vi "Autonomous Independent.vi"() -> ()   [LabVIEW 2016]
doc: "This VI is called when autonomous begins, and will automatically be terminated when autonomous ends. You can carry out timed or sensor driven robot movement independently without needing to return to the caller."
uses:
  <vilib>/Rock Robotics/WPI/ThirdParty/CanMotor/TalonSRX/WPI_CANTalonSRX_APIControlMode.ctl
  Auton.ctl
  AutonEncCounts.ctl
  <vilib>/Rock Robotics/WPI/Relay/WPI_RelayValue.ctl
  <vilib>/Rock Robotics/Network Tables/NT Read String.vi
  <vilib>/Rock Robotics/Network Tables/NT Write String.vi
  <vilib>/Rock Robotics/Network Tables/NT Write Number.vi
panel:
  out "ElapsedTime":u32
  # "Be sure to right-click and choose Data Operations>>Make Current Value default if you want to save the array values with the VI"
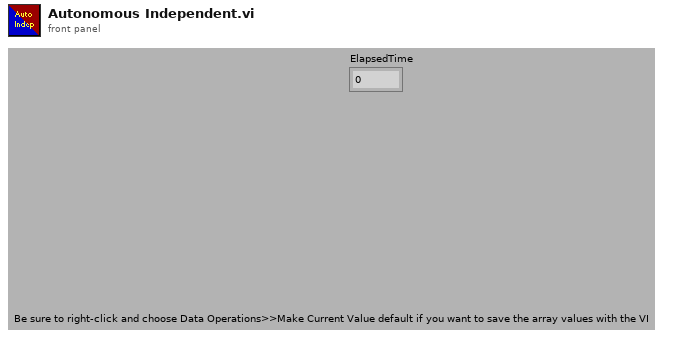
[diagram p1: front panel]
types:
  T1 = enum16{"Integer", "Float", "Boolean", "Enum", "String", "Close"}
  T2 = typedef "Auton.ctl" = enum16{"VisionTarget", "Wait", "Initialize", "Stop", "Reset", "StraightForward", "StraightBack", "SolenoidControl", "SharpLeftCurve", "SharpRightCurve", "GradLeftCurve", "GradRightCurve", "TurnLeft90", "TurnRight90", "TurnLeft60", "TurnRight60", "TurnLeft45", "TurnRight45", "Shoot", "SpinUp", "GearApproach", "ShortShoot", "SlowForward", "TimeForward", "Pause", "HopperDrive"}
  T3 = typedef "AutonEncCounts.ctl" = i32
  T4 = cluster{"Action":T2[], "EncoderCounts":T3[], "GearLift":bool[], "FuelFlap":bool[]}
  T5 = cluster{"Action":T2[], T3[], "GearLift":bool[], "FuelFlap":bool[]}
  T6 = typedef "WPI_MotorControlDeviceRef.ctl" = cluster{"DeviceStatus":errorcluster, "Type":T7, "PWM":cluster{"PWM Channel":T8, "DeadBand":T9}, "CAN":cluster{"Device Number":u8, "SetOutput VI Ref":variant, "GetOutput VI Ref":variant, "Enable VI Ref":variant, "Disable VI Ref":variant, "Data":variant}, "Invert":bool}
  T7 = typedef "WPI_MotorControlType.ctl" = enum16{"PWM", "CAN"}
  T8 = typedef "FPGA_DIOPWMChannel.ctl" = enum8{"PWM 0", "PWM 1", "PWM 2", "PWM 3", "PWM 4", "PWM 5", "PWM 6", "PWM 7", "PWM 8", "PWM 9", "PWM MXP 0", "PWM MXP 1", "PWM MXP 2", "PWM MXP 3", "PWM MXP 4", "PWM MXP 5", "PWM MXP 6", "PWM MXP 7", "PWM MXP 8", "PWM MXP 9", "Invalid"}
  T9 = typedef "WPI_PWMDeadband.ctl" = cluster{"Name":string, "maxPositivePwm":i32, "minPositivePwm":i32, "centerPwm":i32, "maxNegativePwm":i32, "minNegativePwm":i32, "angularRange":u16}
  T10 = enum16{"Integer", "Float", "Boolean", "Enum", "String"}
  T11 = typedef "WPI_CANTalonSRX_APIControlMode.ctl" = enum8{"Percent VBus", "Speed", "Position", "Slave", "Unchanged / Invalid", "Voltage Compensation", "Current", "Motion Profile", "Motion Magic"}
  T12 = typedef "WPI_RelayValue.ctl" = enum16{"Off", "On", "Forward", "Reverse"}
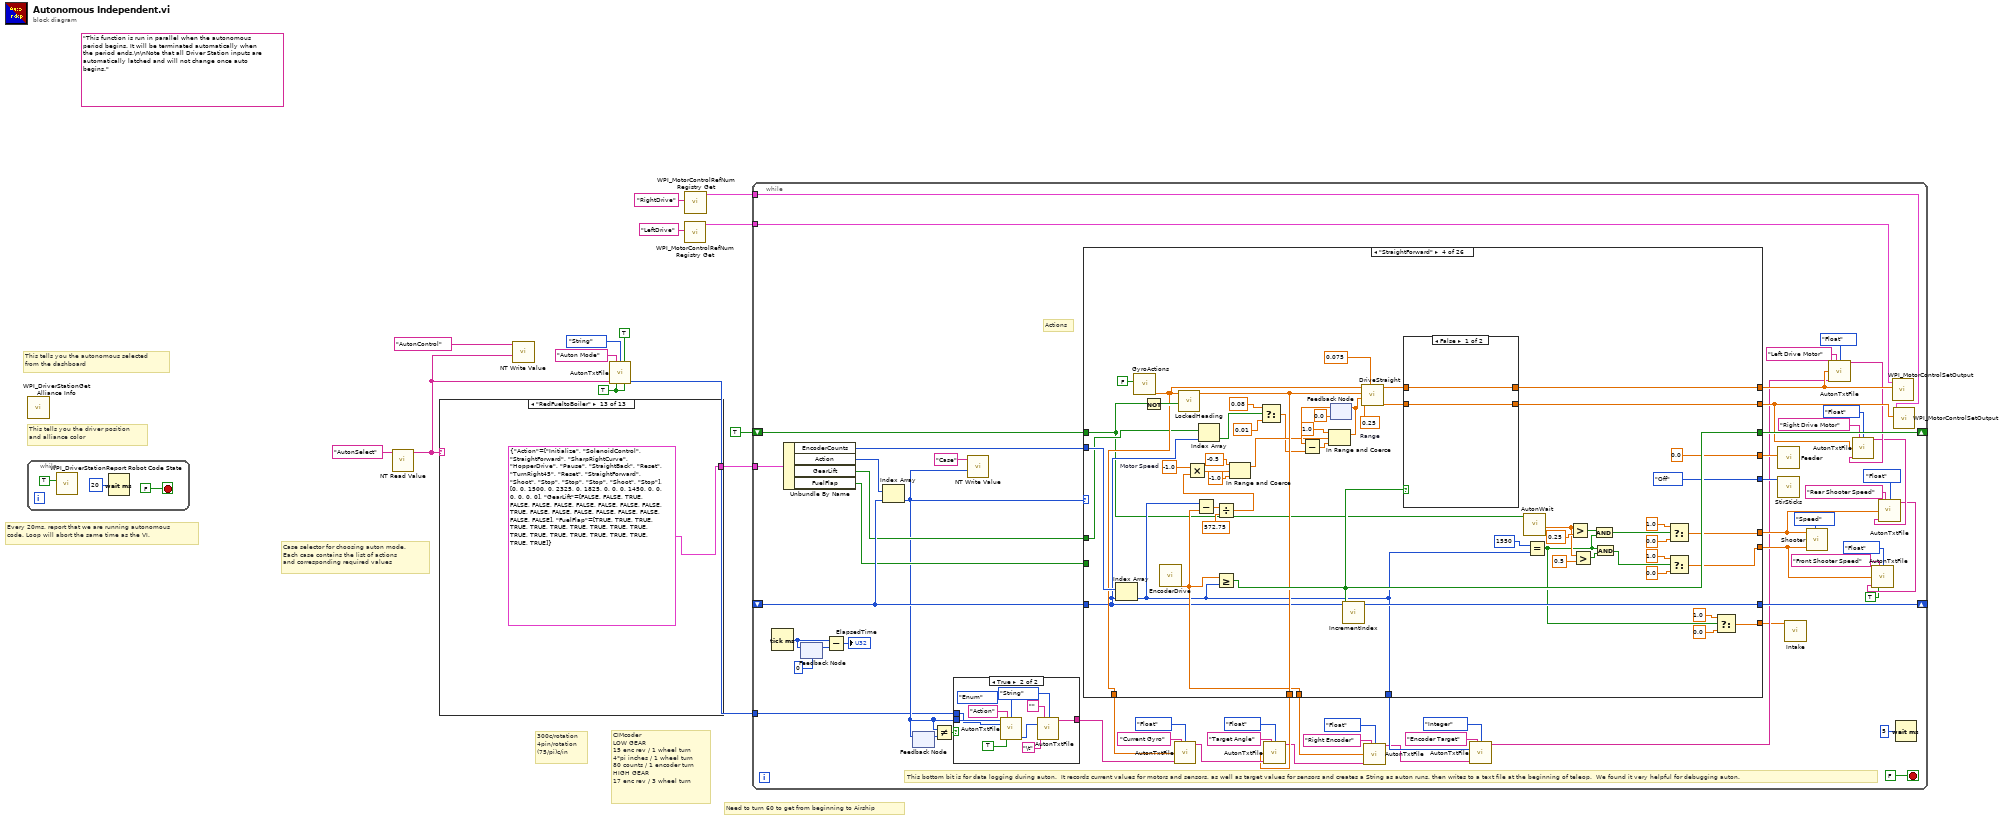
[diagram p0: block diagram]
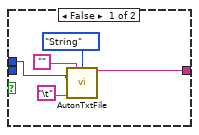
[diagram p2: hidden frame]
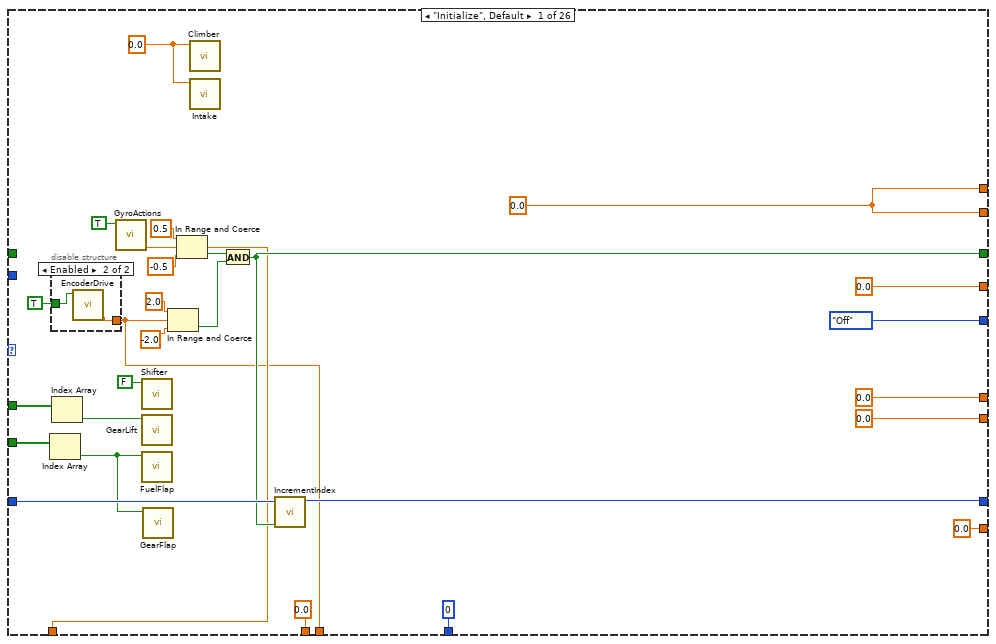
[diagram p3: hidden frame]
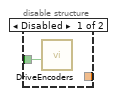
[diagram p4: hidden frame]
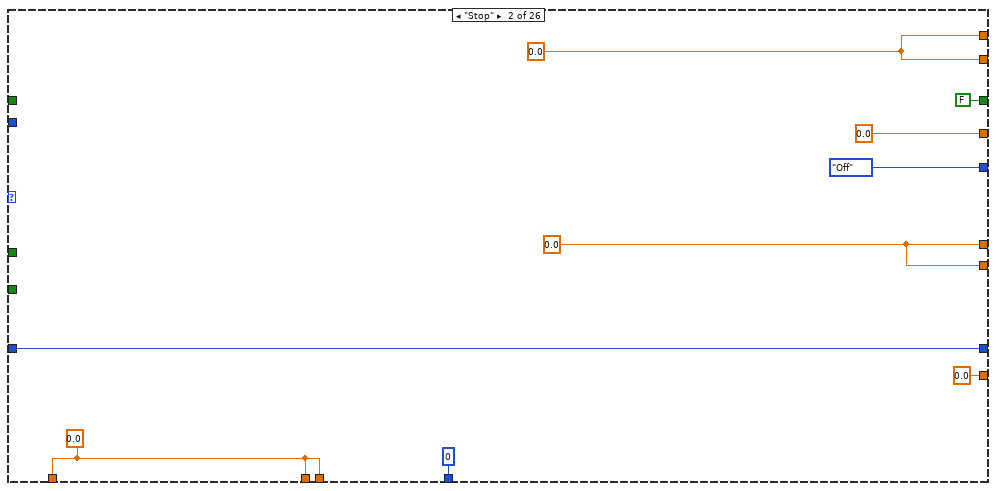
[diagram p5: hidden frame]
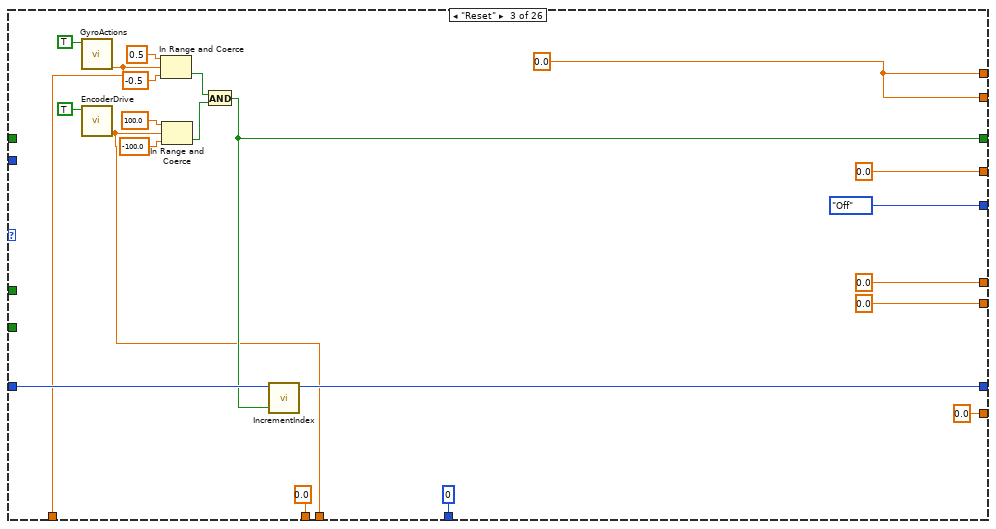
[diagram p6: hidden frame]
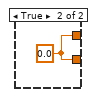
[diagram p7: hidden frame]
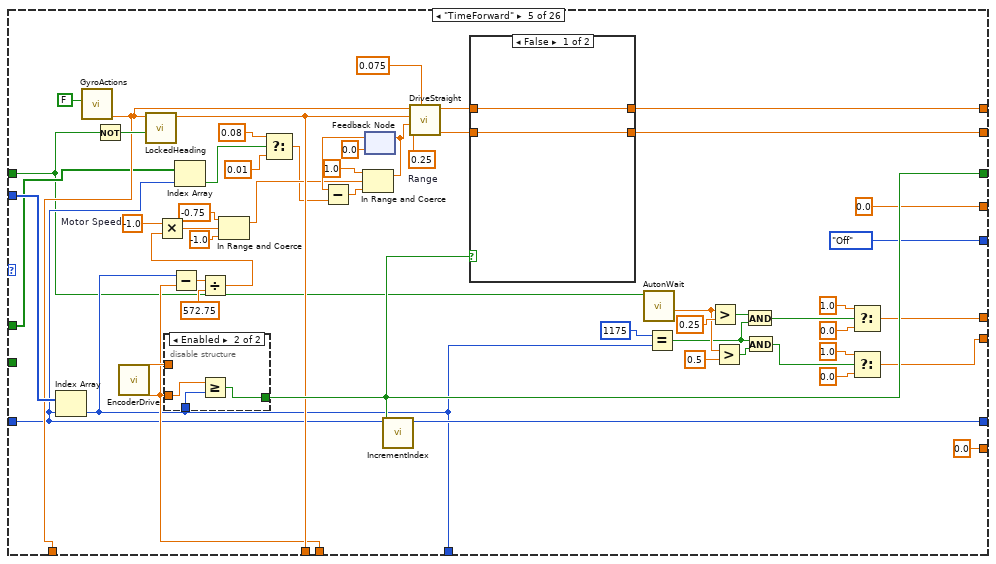
[diagram p8: hidden frame]
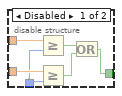
[diagram p9: hidden frame]
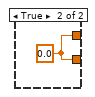
[diagram p10: hidden frame]
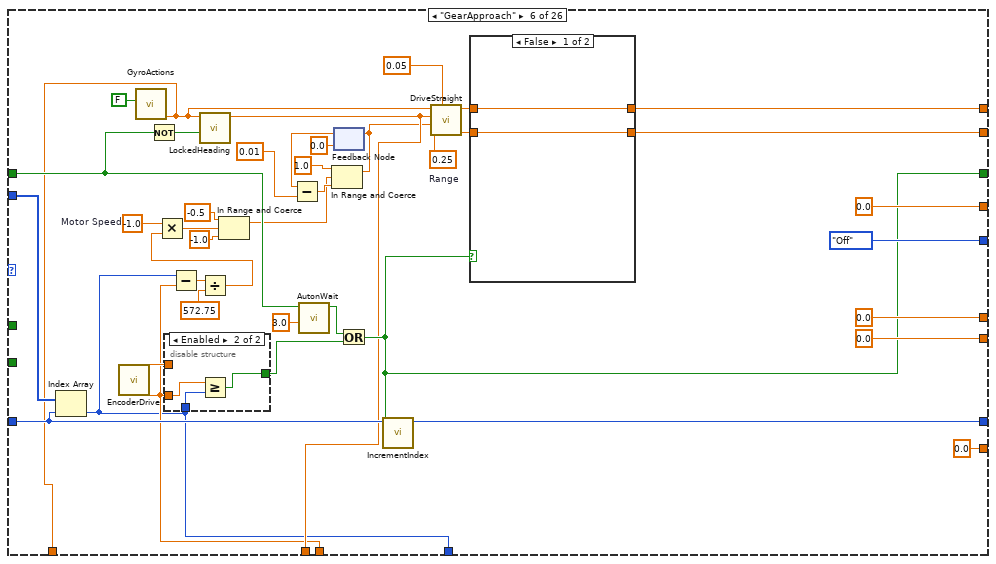
[diagram p11: hidden frame]
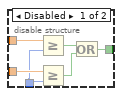
[diagram p12: hidden frame]
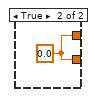
[diagram p13: hidden frame]
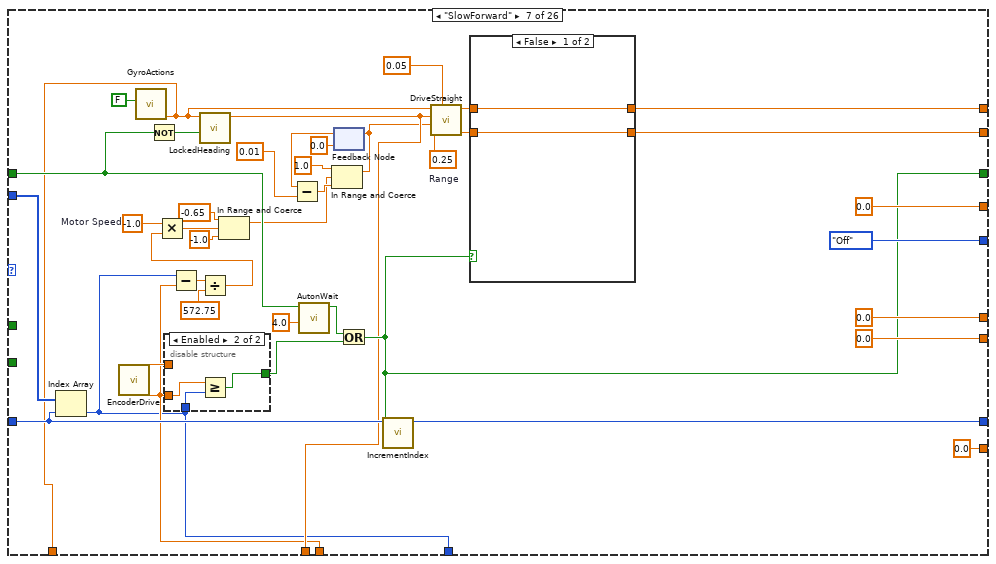
[diagram p14: hidden frame]
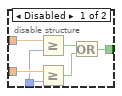
[diagram p15: hidden frame]
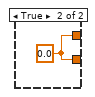
[diagram p16: hidden frame]
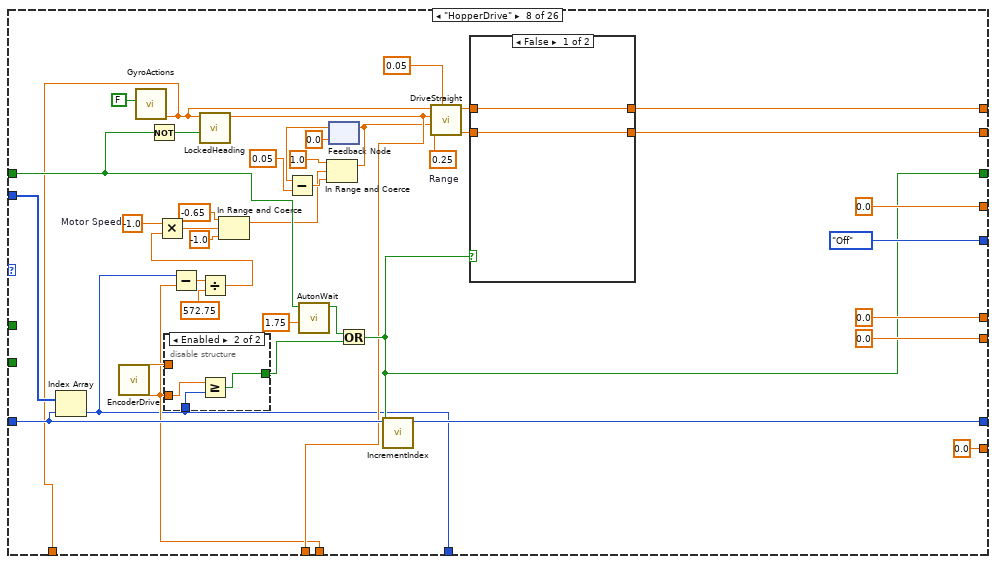
[diagram p17: hidden frame]
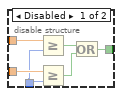
[diagram p18: hidden frame]
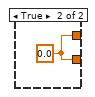
[diagram p19: hidden frame]
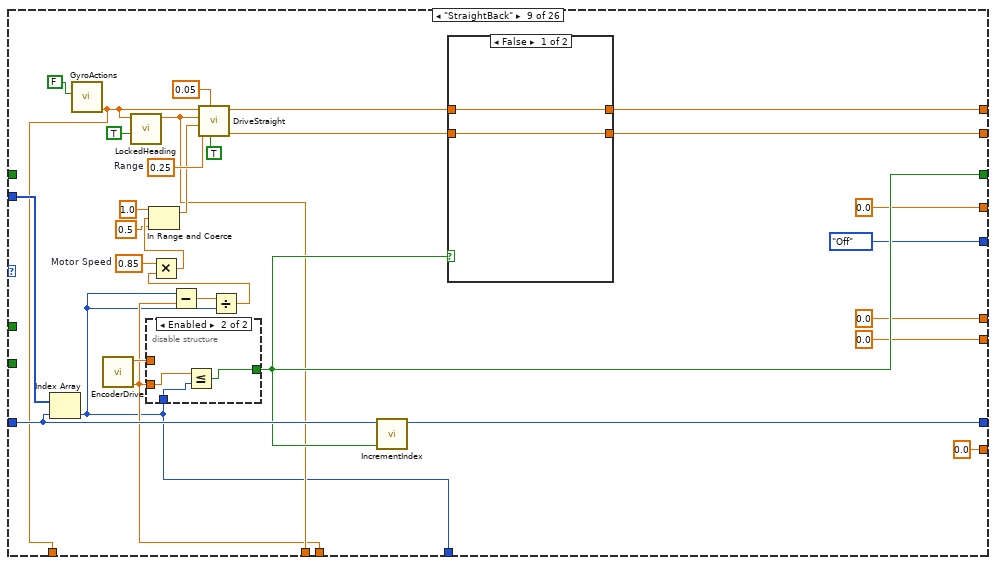
[diagram p20: hidden frame]
diagram:
  w4 = TRUE ("writeToFile?")
  (unwired) "This function is run in parallel when the autonomous period begins. It will be terminated automatically when the period ends.\n\nNote that all Driver Station inputs are automatically latched and will not change once auto begins."
  # "Case selector for choosing auton mode.\nEach case contains the list of actions\nand corresponding required values"
  # "300c/rotation\n4pin/rotation\n(75/pi)c/in"
  # "CIMcoder\nLOW GEAR\n15 enc rev / 1 wheel turn\n4*pi inches / 1 wheel turn\n80 counts / 1 encoder turn\nHIGH GEAR\n17 enc rev / 3 wheel turn"
  # "Need to turn 60 to get from beginning to Airship"
  # "This tells you the autonomous selected\nfrom the dashboard"
  # "Every 20ms, report that we are running autonomous\ncode. Loop will abort the same time as the VI."
  # "This tells you the driver position\nand alliance color"
  n1 = while {
    stop <- FALSE stop-if-true
    n2 = call <vilib>:"WPI_DriverStationReport Robot Code State.vi"("Autonomous"=TRUE) -> ()  [unwired: 10 in, 1 out]
    n3 = Wait (ms)(milliseconds to wait=u32 20) -> ()  [unwired: 1 out]
  }
  n4 = call <vilib>:"WPI_DriverStationGet Alliance Info.vi"() -> ()  [unwired: 12 out]
  n5 = call-poly <vilib>:"NT Read Value.vi"("Name"="AutonSelect") -> ("String"=w2:string)  [unwired: 9 in, 1 out]
  n6 = case shown="\"RedFueltoBoiler\"" w2 {
    tunnel: [T4 {"Action"=[enum."Stop", enum."StraightForward", enum."StraightBack", enum."TurnLeft90", enum."Reset", enum."TurnRight60", enum."TurnRight60", enum."TurnLeft90"], "EncoderCounts"=[0, 0, 0, 0, 0, 0, 0, 0], "GearLift"=[FALSE, TRUE, TRUE, TRUE, TRUE, TRUE, TRUE, TRUE, TRUE, TRUE, TRUE], "FuelFlap"=[FALSE, TRUE, TRUE, TRUE, TRUE, TRUE, TRUE, TRUE, TRUE, TRUE, TRUE]} T4 {"Action"=[enum."Initialize", enum."StraightForward", enum."Stop", enum."TurnLeft90", enum."Reset", enum."TurnRight60", enum."TurnRight60", enum."TurnLeft90"], "EncoderCounts"=[0, 2291, 0, 0, 0, 0, 0, 0], "GearLift"=[FALSE, FALSE, FALSE, TRUE, TRUE, TRUE, TRUE, TRUE, TRUE, TRUE, TRUE], "FuelFlap"=[FALSE, FALSE, FALSE, TRUE, TRUE, TRUE, TRUE, TRUE, TRUE, TRUE, TRUE]} T4 {"Action"=[enum."Initialize", enum."ShortShoot", enum."Reset", enum."TurnRight90", enum."StraightForward", enum."Stop", enum."TurnRight60", enum."TurnLeft90"], "EncoderCounts"=[0, 0, 0, 0, 2500, 0, 0, 0], "GearLift"=[FALSE, FALSE, FALSE, FALSE, FALSE, FALSE, TRUE, TRUE, TRUE, TRUE, TRUE], "FuelFlap"=[FALSE, FALSE, FALSE, FALSE, FALSE, FALSE, FALSE, FALSE, TRUE, TRUE, TRUE]} T4 {"Action"=[enum."Initialize", enum."ShortShoot", enum."Reset", enum."TurnLeft90", enum."StraightForward", enum."Stop", enum."TurnRight60", enum."TurnLeft90"], "EncoderCounts"=[0, 0, 0, 0, 2500, 0, 0, 0], "GearLift"=[FALSE, FALSE, FALSE, FALSE, FALSE, FALSE, TRUE, TRUE, TRUE, TRUE, TRUE], "FuelFlap"=[FALSE, FALSE, FALSE, FALSE, FALSE, FALSE, FALSE, FALSE, TRUE, TRUE, TRUE]} T4 {"Action"=[enum."Initialize", enum."SpinUp", enum."Shoot", enum."Stop", enum."StraightForward", enum."Stop", enum."TurnRight60", enum."TurnLeft90"], "EncoderCounts"=[0, 0, 0, 0, 0, 0, 0, 0], "GearLift"=[FALSE, FALSE, FALSE, FALSE, TRUE, TRUE, TRUE, TRUE, TRUE, TRUE, TRUE], "FuelFlap"=[FALSE, FALSE, FALSE, FALSE, FALSE, FALSE, FALSE, FALSE, TRUE, TRUE, TRUE]} T4 {"Action"=[enum."Initialize", enum."StraightForward", enum."Reset", enum."TurnLeft60", enum."Reset", enum."GearApproach", enum."SolenoidControl", enum."Pause", enum."StraightBack", enum."Reset", enum."TurnRight60", enum."Reset", enum."StraightForward", enum."Stop"], "EncoderCounts"=[0, 1550, 0, 0, 0, 1650, 0, 0, 500, 0, 0, 0, 7000, 0], "GearLift"=[FALSE, FALSE, FALSE, FALSE, FALSE, FALSE, TRUE, FALSE, FALSE, FALSE, FALSE, FALSE, FALSE, FALSE], "FuelFlap"=[FALSE, FALSE, FALSE, FALSE, FALSE, FALSE, FALSE, FALSE, FALSE, FALSE, FALSE, FALSE, FALSE, FALSE]} T4 {"Action"=[enum."Initialize", enum."StraightForward", enum."Reset", enum."TurnRight60", enum."Reset", enum."StraightForward", enum."SolenoidControl", enum."Pause", enum."StraightBack", enum."Reset", enum."TurnLeft60", enum."Reset", enum."StraightForward", enum."Stop"], "EncoderCounts"=[0, 1550, 0, 0, 0, 1650, 0, 0, 500, 0, 0, 0, 7000, 0], "GearLift"=[FALSE, FALSE, FALSE, FALSE, FALSE, FALSE, TRUE, FALSE, FALSE, FALSE, FALSE, FALSE, FALSE, FALSE], "FuelFlap"=[FALSE, FALSE, FALSE, FALSE, FALSE, FALSE, FALSE, FALSE, FALSE, FALSE, FALSE, FALSE, FALSE, FALSE]} T4 {"Action"=[enum."Initialize", enum."SlowForward", enum."SolenoidControl", enum."Pause", enum."StraightBack", enum."Stop", enum."TurnRight60", enum."TurnLeft90"], "EncoderCounts"=[0, 1650, 0, 0, 1000, 0, 0, 0], "GearLift"=[FALSE, FALSE, TRUE, FALSE, FALSE, FALSE, TRUE, TRUE, TRUE, TRUE, TRUE], "FuelFlap"=[FALSE, FALSE, FALSE, FALSE, FALSE, FALSE, TRUE, TRUE, TRUE, TRUE, TRUE]} T4 {"Action"=[enum."Initialize", enum."StraightForward", enum."Reset", enum."TurnRight60", enum."Reset", enum."GearApproach", enum."SolenoidControl", enum."Pause", enum."StraightBack", enum."Reset", enum."TurnLeft60", enum."Reset", enum."StraightForward", enum."Stop"], "EncoderCounts"=[0, 1550, 0, 0, 0, 1845, 0, 0, 929, 0, 0, 0, 7000, 0], "GearLift"=[FALSE, FALSE, FALSE, FALSE, FALSE, FALSE, TRUE, FALSE, FALSE, FALSE, FALSE, FALSE, FALSE], "FuelFlap"=[FALSE, FALSE, FALSE, FALSE, FALSE, FALSE, FALSE, FALSE, FALSE, FALSE, FALSE, FALSE, FALSE]} T4 {"Action"=[enum."Initialize", enum."StraightForward", enum."Reset", enum."TurnLeft60", enum."Reset", enum."StraightForward", enum."SolenoidControl", enum."StraightBack", enum."Reset", enum."TurnRight60", enum."Reset", enum."StraightForward", enum."Stop"], "EncoderCounts"=[0, 1471, 0, 0, 0, 1645, 0, 929, 0, 0, 0, 7000, 0], "GearLift"=[FALSE, FALSE, FALSE, FALSE, FALSE, FALSE, TRUE, FALSE, FALSE, FALSE, FALSE, FALSE, FALSE, FALSE], "FuelFlap"=[FALSE, FALSE, FALSE, FALSE, FALSE, FALSE, FALSE, FALSE, FALSE, FALSE, FALSE, FALSE, FALSE]} T5 {"Action"=[enum."Initialize", enum."SolenoidControl", enum."StraightForward", enum."SharpLeftCurve", enum."HopperDrive", enum."Pause", enum."StraightBack", enum."Reset", enum."TurnLeft45", enum."Reset", enum."StraightForward", enum."Shoot", enum."Stop", enum."Stop", enum."Stop", enum."Shoot", enum."Stop"], [0, 0, 1500, 0, 3475, 0, 2935, 0, 0, 0, 1450, 0, 0, 0, 0, 0, 0], "GearLift"=[FALSE, FALSE, TRUE, FALSE, FALSE, FALSE, FALSE, FALSE, FALSE, FALSE, TRUE, FALSE, FALSE, FALSE, FALSE, FALSE, FALSE, FALSE, FALSE], "FuelFlap"=[TRUE, TRUE, TRUE, TRUE, TRUE, TRUE, TRUE, TRUE, TRUE, TRUE, TRUE, TRUE, TRUE, TRUE, TRUE, TRUE, TRUE, TRUE, TRUE]} T4 {"Action"=[enum."Initialize", enum."TimeForward", enum."Stop", enum."TurnLeft90", enum."Reset", enum."TurnRight60", enum."TurnRight60", enum."TurnLeft90"], "EncoderCounts"=[0, 0, 0, 0, 0, 0, 0, 0], "GearLift"=[FALSE, FALSE, FALSE, TRUE, TRUE, TRUE, TRUE, TRUE, TRUE, TRUE, TRUE], "FuelFlap"=[FALSE, FALSE, FALSE, TRUE, TRUE, TRUE, TRUE, TRUE, TRUE, TRUE, TRUE]} T5 {"Action"=[enum."Initialize", enum."SolenoidControl", enum."StraightForward", enum."SharpRightCurve", enum."HopperDrive", enum."Pause", enum."StraightBack", enum."Reset", enum."TurnRight45", enum."Reset", enum."StraightForward", enum."Shoot", enum."Stop", enum."Stop", enum."Stop", enum."Shoot", enum."Stop"], [0, 0, 1500, 0, 2325, 0, 1825, 0, 0, 0, 1450, 0, 0, 0, 0, 0, 0], "GearLift"=[FALSE, FALSE, TRUE, FALSE, FALSE, FALSE, FALSE, FALSE, FALSE, FALSE, TRUE, FALSE, FALSE, FALSE, FALSE, FALSE, FALSE, FALSE, FALSE], "FuelFlap"=[TRUE, TRUE, TRUE, TRUE, TRUE, TRUE, TRUE, TRUE, TRUE, TRUE, TRUE, TRUE, TRUE, TRUE, TRUE, TRUE, TRUE, TRUE, TRUE]}] -> w11
    frame "DoNothing", Default {
    }
    frame "CrossLine" {
    }
    frame "BlueShootAndCross" {
    }
    frame "RedShootAndCross" {
    }
    frame "JustShoot" {
    }
    frame "BlueGearRight" {
      # "603"
    }
    frame "RedGearLeft" {
    }
    frame "GearStraight" {
    }
    frame "BlueGearLeft" {
    }
    frame "RedGearRight" {
    }
    frame "BlueFueltoBoiler" {
    }
    frame "TimedForward" {
    }
    frame "RedFueltoBoiler" {
    }
  }
  n7 = call-poly <vilib>:"NT Write Value.vi"("String"=w2, "Name"="AutonControl") -> ()  [unwired: 9 in, 1 out]
  n8 = call "AutonTxtFile.vi"("dataName"="Auton Mode", "mode"=T1."String", "reset?"=TRUE, "string"=w2, "newLine?"=w4, "doubleSpace?"=w4) -> ("flowControl2"=w1:i32)  [unwired: 8 in, 1 out]
  n9 = call <vilib>:"WPI_MotorControlRefNum Registry Get.vi"("refnum name"="LeftDrive") -> ("MotorControlDevRef"=w10:T6)  [unwired: 9 in, 1 out]
  n10 = call <vilib>:"WPI_MotorControlRefNum Registry Get.vi"("refnum name"="RightDrive") -> ("MotorControlDevRef"=w9:T6)  [unwired: 9 in, 1 out]
  n11 = while {
    shift-right: [w87] -> _
    shift-left: _ -> [w86]
    shift-right: [w84] -> _
    shift-left: TRUE -> [w85]
    tunnel: w11 -> [w76]
    tunnel: w10 -> [w75]
    tunnel: w9 -> [w74]
    tunnel: w1 -> [w33]
    stop <- FALSE stop-if-true
    # "This bottom bit is for data logging during auton.  It records current values for motors and sensors, as well as target values for sensors and creates a String as auton runs, then writes to a text file at the beginning of teleop.  We found it very helpful for debugging auton."
    # "Actions"
    n12 = Tick Count (ms)() -> (millisecond timer value=w72:u32)
    n13 = Unbundle By Name(w76) -> ("EncoderCounts"=w81:T3[], "Action"=w80:T2[], "GearLift"=w83:bool[], "FuelFlap"=w82:bool[])
    n14 = feedback-in #1(w72) -> ()
    n15 = feedback #1(u32 0 ("millisecond timer value")) -> (w73:u32)
    n16 = Subtract(x=w72, y=w73) -> (x-y=→"ElapsedTime":u32)
    n17 = Index Array(array=w80, index=w86) -> (element=w67:T2)
    n18 = feedback-in #2(w67) -> ()
    n19 = feedback #2() -> (w68:T2)  [unwired: 1 in]
    n20 = Not Equal?(x=w67, y=w68) -> (x != y?=w66:bool)
    n21 = case shown="True" w66 {
      tunnel: w67 -> [_ w102]
      tunnel: [w91 w99] -> w32
      tunnel: w33 -> [w90 w100]
      frame False {
        n22 = call "AutonTxtFile.vi"("dataName"="", "mode"=T10."String", "integer"=w90, "string"="\t") -> ("flowControl"=w91:string)  [unwired: 10 in, 1 out]
      }
      frame True {
        n23 = call "AutonTxtFile.vi"("enum"=w102, "dataName"="Action", "mode"=T10."Enum", "integer"=w100, "newLine?"=TRUE) -> ("flowControl2"=w98:i32)  [unwired: 9 in, 1 out]
        n24 = call "AutonTxtFile.vi"("dataName"="", "mode"=T10."String", "integer"=w98, "string"="\t") -> ("flowControl"=w99:string)  [unwired: 10 in, 1 out]
      }
    }
    n25 = call-poly <vilib>:"NT Write Value.vi"("Numeric"=w67, "Name"="Case") -> ()  [unwired: 9 in, 1 out]
    n26 = case shown="\"StraightForward\"" w67 {
      tunnel: [w130 w142 w162 w219 w276 w328 w380 w432 w472 w501 w513 w526 w538 w556 w580 w598 w612 w628 w646 w664 w682 w698 w714 w725 w740 w838] -> w87
      tunnel: [w110 w143 w164 w194 w250 w292 w344 w395 w465 w497 w509 w522 w536 0.0 ("Power") w572 w590 w608 w626 w644 w662 w684 w700 w716 w723 w746 w836] -> w63
      tunnel: [w110 w143 w164 w191 w247 w291 w343 w394 w464 w497 w509 w522 w535 w554 w571 0.0 ("Power") w607 w625 w643 w661 w684 w700 w716 w723 w745 w836] -> w60
      tunnel: w81 -> [_ _ _ w216 w273 w325 w377 w429 w471 _ _ _ _ _ _ _ _ _ _ _ _ _ _ _ _ w831]
      tunnel: w86 -> [w131 w142 w163 w184 w240 w324 w376 w428 w470 w496 w514 w527 w539 w557 w579 w597 w613 w629 w647 w665 w683 w699 w715 w726 w741 w830]
      tunnel: w85 -> [_ _ _ w179 w235 w299 w351 w403 _ w495 w512 w525 w540 w558 w581 w599 w611 w630 w648 w666 w680 w696 w712 w728 w739 w839]
      tunnel: [w111 FALSE ("Completed") w153 w213 w269 w300 w352 w404 w463 w495 w512 w525 w541 w559 w578 w596 w610 w631 w649 w667 w679 w691 w711 w724 w742 w837] -> w84
      tunnel: w83 -> [w129 _ _ w185 w241 _ _ _ _ w500 _ _ _ _ _ _ _ _ _ _ _ _ _ _ _ _]
      tunnel: w82 -> [w128 _ _ _ _ _ _ _ _ w499 _ _ _ _ _ _ _ _ _ _ _ _ _ _ _ _]
      tunnel: [0.0 ("RearMotorIn") w141 0.0 ("RearMotorIn") w186 w242 0.0 ("RearMotorIn") 0.0 ("RearMotorIn") 0.0 ("RearMotorIn") 0.0 ("RearMotorIn") 0.0 ("RearMotorIn") w507 w520 w534 w553 w570 w589 w606 w624 w642 w660 1.0 ("f") 0.8 ("RearMotorIn") w710 w722 0.8 ("RearMotorIn") w824] -> w53
      tunnel: [0.0 ("RearMotorIn") w141 0.0 ("RearMotorIn") w169 w224 0.0 ("RearMotorIn") 0.0 ("RearMotorIn") 0.0 ("RearMotorIn") 0.0 ("RearMotorIn") 0.0 ("RearMotorIn") w507 w520 w534 w553 w570 w589 w606 w624 w642 w660 0.95 ("RearMotorIn") 0.95 ("RearMotorIn") w710 w722 0.95 ("RearMotorIn") w824] -> w51
      tunnel: [0.0 ("Power") 0.0 ("Power") 0.0 ("Power") 0.0 ("Power") 0.0 ("Power") 0.0 ("Power") 0.0 ("Power") 0.0 ("Power") 0.0 ("Power") 0.0 ("Power") w507 w520 w534 w553 w570 w589 w606 w624 w642 w660 1.0 ("RearMotorIn") w695 0.0 ("Power") 0.0 ("RearMotorIn") w744 0.0 ("Power")] -> w78
      tunnel: [WPI_RelayValue."Off" ("RelayValue") WPI_RelayValue."Off" ("RelayValue") WPI_RelayValue."Off" ("RelayValue") WPI_RelayValue."Off" ("RelayValue") WPI_RelayValue."Off" ("RelayValue") WPI_RelayValue."Off" ("RelayValue") WPI_RelayValue."Off" ("RelayValue") WPI_RelayValue."Off" ("RelayValue") WPI_RelayValue."Off" ("RelayValue") WPI_RelayValue."Off" ("RelayValue") WPI_RelayValue."Off" ("RelayValue") WPI_RelayValue."Off" ("RelayValue") WPI_RelayValue."Off" ("RelayValue") WPI_RelayValue."Off" ("RelayValue") WPI_RelayValue."Off" ("RelayValue") WPI_RelayValue."Off" ("RelayValue") WPI_RelayValue."Off" ("RelayValue") WPI_RelayValue."Off" ("RelayValue") WPI_RelayValue."Off" ("RelayValue") WPI_RelayValue."Off" ("RelayValue") WPI_RelayValue."Forward" ("RelayValue") w694 WPI_RelayValue."Off" ("RelayValue") WPI_RelayValue."Off" ("RelayValue") w743 WPI_RelayValue."Off" ("RelayValue")] -> w77
      tunnel: [w109 w137 w148 w196 w252 w297 w349 w401 w450 w489 w505 w518 w532 w551 w568 w587 w604 w622 w640 w658 w674 w687 w707 w719 w733 w833] -> w48
      tunnel: [w108 w137 w147 w195 w251 w295 w347 w399 w448 w489 w504 w517 0.0 ("Yaw") 0.0 ("Yaw") 0.0 ("Yaw") 0.0 ("Yaw") 0.0 ("Yaw") 0.0 ("Yaw") 0.0 ("Yaw") 0.0 ("Yaw") w674 w687 w707 w719 0.0 ("Yaw") w833] -> w45
      tunnel: [0.0 ("LockedHeading") w137 0.0 ("LockedHeading") w197 w253 w296 w348 w400 w449 w489 w504 w517 w531 w550 w567 w586 w603 w621 w639 w657 w674 w687 w707 w719 w732 w833] -> w39
      tunnel: [T3 0 ("EncCounts") T3 0 ("EncCounts") T3 0 ("EncCounts") w190 w246 w294 w346 w398 w447 T3 0 ("EncCounts") T3 0 ("EncCounts") T3 0 ("EncCounts") T3 0 ("EncCounts") T3 0 ("EncCounts") T3 0 ("EncCounts") T3 0 ("EncCounts") T3 0 ("EncCounts") T3 0 ("EncCounts") T3 0 ("EncCounts") T3 0 ("EncCounts") T3 0 ("EncCounts") T3 0 ("EncCounts") T3 0 ("EncCounts") T3 0 ("EncCounts") T3 0 ("EncCounts") T3 0 ("EncCounts")] -> w37
      tunnel: [0.0 ("f") 0.0 ("f") 0.0 ("f") w166 0.0 ("f") 0.0 ("f") 0.0 ("f") 0.0 ("f") 0.0 ("f") 0.0 ("f") 0.0 ("f") 0.0 ("f") 0.0 ("f") 0.0 ("f") 0.0 ("f") 0.0 ("f") 0.0 ("f") 0.0 ("f") 0.0 ("f") 0.0 ("f") 1.0 ("f") 1.0 ("f") 0.0 ("f") 0.0 ("f") 0.0 ("f") 0.0 ("f")] -> w31
      frame "Initialize", Default {
        w125 = 0.0 ("Power")
        w110 = 0.0 ("Left")
        n27 = Index Array(array=w128) -> (element=w123:bool)  [unwired: 1 in]
        n28 = disable-structure shown="Enabled" {
          disable-tunnel: TRUE ("Reset?") -> [w132 w134]
          disable-tunnel: [_ w133] -> w108
          frame Disabled {
            n29 = call "DriveEncoders.vi"("Reset?"=w132) -> ()  [unwired: 9 in, 2 out]
          }
          frame Enabled {
            n30 = call "EncoderDrive.vi"("Reset?"=w134) -> ("RightEncder"=w133:dbl)  [unwired: 9 in, 1 out]
          }
        }
        n31 = Index Array(array=w129) -> (element=w127:bool)  [unwired: 1 in]
        n32 = call "GyroActions.vi"("Zero"=TRUE) -> ("Yaw"=w109:dbl)  [unwired: 9 in, 1 out]
        n33 = call "Shifter.vi"("Shift"=FALSE) -> ()  [unwired: 11 in]
        n34 = call "GearLift.vi"("Gear Up"=w127) -> ()  [unwired: 11 in]
        n35 = call "FuelFlap.vi"("Fuel Flap"=w123) -> ()  [unwired: 11 in]
        n36 = call "GearFlap.vi"("Gear Flap"=w123) -> ()  [unwired: 11 in]
        n37 = In Range and Coerce(upper limit=2.0, x=w108, lower limit=-2.0) -> (In Range?=w112:bool)  [unwired: 1 out]
        n38 = In Range and Coerce(upper limit=0.5, x=w109, lower limit=-0.5) -> (In Range?=w113:bool)  [unwired: 1 out]
        n39 = call "Climber.vi"("Power"=w125) -> ()  [unwired: 11 in]
        n40 = call "Intake.vi"("Power"=w125) -> ()  [unwired: 11 in]
        n41 = And(x=w113, y=w112) -> (x .and. y?=w111:bool)
        n42 = call "IncrementIndex.vi"("Increment?"=w111, "IndexIn"=w131) -> ("IndexOut"=w130:i32)  [unwired: 9 in]
      }
      frame "Stop" {
        w137 = 0.0 ("Yaw")
        w141 = 0.0 ("RearMotorIn")
        w143 = 0.0 ("Left")
      }
      frame "Reset" {
        w164 = 0.0 ("Left")
        n43 = call "GyroActions.vi"("Zero"=TRUE) -> ("Yaw"=w148:dbl)  [unwired: 9 in, 1 out]
        n44 = call "EncoderDrive.vi"("Reset?"=TRUE ("Boolean")) -> ("RightEncder"=w147:dbl)  [unwired: 9 in, 1 out]
        n45 = In Range and Coerce(upper limit=0.5, x=w148, lower limit=-0.5) -> (In Range?=w154:bool)  [unwired: 1 out]
        n46 = In Range and Coerce(upper limit=100.0, x=w147, lower limit=-100.0) -> (In Range?=w155:bool)  [unwired: 1 out]
        n47 = And(x=w154, y=w155) -> (x .and. y?=w153:bool)
        n48 = call "IncrementIndex.vi"("Increment?"=w153, "IndexIn"=w163) -> ("IndexOut"=w162:i32)  [unwired: 9 in]
      }
      frame "StraightForward" {
        w218 = 0.25  # Range
        w211 = -1.0  # Motor Speed
        n49 = Index Array(array=w216, index=w184) -> (element=w190:T3)
        n50 = call "GyroActions.vi"("Update?"=FALSE) -> ("Yaw"=w196:dbl)  [unwired: 9 in, 1 out]
        n51 = Not(x=w179) -> (.not. x?=w212:bool)
        n52 = call "EncoderDrive.vi"() -> ("RightEncder"=w195:dbl)  [unwired: 10 in, 1 out]
        n53 = call "LockedHeading.vi"("LockHeading"=w212, "Heading In"=w196) -> ("LockedHeading"=w197:dbl)  [unwired: 9 in]
        n54 = Subtract(x=w190, y=w195) -> (x-y=w210:dbl)
        n55 = Index Array(array=w185, index=w184) -> (element=w182:bool)
        n56 = Divide(x=w210, y=572.75) -> (x/y=w209:dbl)
        n57 = Multiply(x=w211, y=w209) -> (x*y=w208:dbl)
        n58 = Greater Or Equal?(x=w195, y=w190) -> (x >= y?=w213:bool)
        n59 = In Range and Coerce(upper limit=-0.5, x=w208, lower limit=-1.0) -> (coerced(x)=w193:dbl)  [unwired: 1 out]
        n60 = Select(t=0.08, s=w182, f=0.01 ("y")) -> (s? t:f=w180:dbl)
        n61 = feedback #3(0.0 ("upper limit")) -> (w199:dbl)
        n62 = Subtract(x=w199, y=w180) -> (x-y=w200:dbl)
        n63 = In Range and Coerce(upper limit=1.0, x=w193, lower limit=w200) -> (coerced(x)=w192:dbl)  [unwired: 1 out]
        n64 = feedback-in #3(w192) -> ()
        n65 = call "IncrementIndex.vi"("Increment?"=w213, "IndexIn"=w184) -> ("IndexOut"=w219:i32)  [unwired: 9 in]
        n66 = call "DriveStraight.vi"("Sensitivity"=0.075, "Range"=w218, "Motor Speed"=w192, "Target"=w197, "Yaw"=w196) -> ("Right"=w215:dbl, "Left"=w214:dbl)  [unwired: 5 in]
        n67 = case shown="False" w213 {
          tunnel: w215 -> [w221 _]
          tunnel: w214 -> [w220 _]
          tunnel: [w221 w222] -> w191
          tunnel: [w220 w222] -> w194
          frame False {
          }
          frame True {
            w222 = 0.0 ("upper limit")
          }
        }
        n68 = call "AutonWait.vi"("First Time?"=w179) -> ("ElapsedTime"=w176:dbl)  [unwired: 9 in, 1 out]
        n69 = Equal?(x=T3 1550, y=w190) -> (x = y?=w165:bool)
        n70 = Greater?(x=w176, y=0.25) -> (0:w175:bool)
        n71 = Greater?(x=w176, y=0.5) -> (0:w174:bool)
        n72 = And(x=w175, y=w165) -> (x .and. y?=w173:bool)
        n73 = And(x=w165, y=w174) -> (x .and. y?=w170:bool)
        n74 = Select(t=1.0, s=w173, f=0.0) -> (s? t:f=w186:dbl)
        n75 = Select(t=1.0, s=w170, f=0.0) -> (s? t:f=w169:dbl)
        n76 = Select(t=1.0, s=w165, f=0.0) -> (s? t:f=w166:dbl)
      }
      frame "TimeForward" {
        w275 = 0.25  # Range
        w267 = -1.0  # Motor Speed
        n77 = Index Array(array=w273, index=w240) -> (element=w246:T3)
        n78 = call "GyroActions.vi"("Update?"=FALSE) -> ("Yaw"=w252:dbl)  [unwired: 9 in, 1 out]
        n79 = Not(x=w235) -> (.not. x?=w268:bool)
        n80 = call "EncoderDrive.vi"() -> ("RightEncder"=w251:dbl, "LeftEncoder"=w270:dbl)  [unwired: 10 in]
        n81 = call "LockedHeading.vi"("LockHeading"=w268, "Heading In"=w252) -> ("LockedHeading"=w253:dbl)  [unwired: 9 in]
        n82 = disable-structure shown="Enabled" {
          disable-tunnel: w251 -> [w282 w285]
          disable-tunnel: w270 -> [w279 _]
          disable-tunnel: [w278 w283] -> w269
          disable-tunnel: w246 -> [w277 w284]
          frame Disabled {
            n83 = Greater Or Equal?(x=w279, y=w277) -> (x >= y?=w281:bool)
            n84 = Greater Or Equal?(x=w282, y=w277) -> (x >= y?=w280:bool)
            n85 = Or(x=w281, y=w280) -> (x .or. y?=w278:bool)
          }
          frame Enabled {
            n86 = Greater Or Equal?(x=w285, y=w284) -> (x >= y?=w283:bool)
          }
        }
        n87 = Subtract(x=w246, y=w251) -> (x-y=w266:dbl)
        n88 = Index Array(array=w241, index=w240) -> (element=w238:bool)
        n89 = Divide(x=w266, y=572.75) -> (x/y=w265:dbl)
        n90 = Multiply(x=w267, y=w265) -> (x*y=w264:dbl)
        n91 = In Range and Coerce(upper limit=-0.75, x=w264, lower limit=-1.0) -> (coerced(x)=w249:dbl)  [unwired: 1 out]
        n92 = Select(t=0.08, s=w238, f=0.01 ("y")) -> (s? t:f=w236:dbl)
        n93 = feedback #4(0.0 ("upper limit")) -> (w255:dbl)
        n94 = Subtract(x=w255, y=w236) -> (x-y=w256:dbl)
        n95 = In Range and Coerce(upper limit=1.0, x=w249, lower limit=w256) -> (coerced(x)=w248:dbl)  [unwired: 1 out]
        n96 = feedback-in #4(w248) -> ()
        n97 = call "IncrementIndex.vi"("Increment?"=w269, "IndexIn"=w240) -> ("IndexOut"=w276:i32)  [unwired: 9 in]
        n98 = call "DriveStraight.vi"("Sensitivity"=0.075, "Range"=w275, "Motor Speed"=w248, "Target"=w253, "Yaw"=w252) -> ("Right"=w272:dbl, "Left"=w271:dbl)  [unwired: 5 in]
        n99 = case shown="False" w269 {
          tunnel: w272 -> [w287 _]
          tunnel: w271 -> [w286 _]
          tunnel: [w287 w288] -> w247
          tunnel: [w286 w288] -> w250
          frame False {
          }
          frame True {
            w288 = 0.0 ("upper limit")
          }
        }
        n100 = call "AutonWait.vi"("First Time?"=w235) -> ("ElapsedTime"=w232:dbl)  [unwired: 9 in, 1 out]
        n101 = Equal?(x=T3 1175, y=w246) -> (x = y?=w230:bool)
        n102 = Greater?(x=w232, y=0.25) -> (0:w231:bool)
        n103 = Greater?(x=w232, y=0.5) -> (0:w229:bool)
        n104 = And(x=w231, y=w230) -> (x .and. y?=w228:bool)
        n105 = And(x=w230, y=w229) -> (x .and. y?=w225:bool)
        n106 = Select(t=1.0, s=w228, f=0.0) -> (s? t:f=w242:dbl)
        n107 = Select(t=1.0, s=w225, f=0.0) -> (s? t:f=w224:dbl)
      }
      frame "GearApproach" {
        w327 = 0.25  # Range
        w319 = -1.0  # Motor Speed
        n108 = Index Array(array=w325, index=w324) -> (element=w294:T3)
        n109 = call "EncoderDrive.vi"() -> ("RightEncder"=w295:dbl, "LeftEncoder"=w321:dbl)  [unwired: 10 in]
        n110 = call "GyroActions.vi"("Update?"=FALSE) -> ("Yaw"=w297:dbl)  [unwired: 9 in, 1 out]
        n111 = Not(x=w299) -> (.not. x?=w320:bool)
        n112 = disable-structure shown="Enabled" {
          disable-tunnel: w295 -> [w334 w337]
          disable-tunnel: w321 -> [w331 _]
          disable-tunnel: [w330 w336] -> w301
          disable-tunnel: w294 -> [w329 w335]
          frame Disabled {
            n113 = Greater Or Equal?(x=w331, y=w329) -> (x >= y?=w333:bool)
            n114 = Greater Or Equal?(x=w334, y=w329) -> (x >= y?=w332:bool)
            n115 = Or(x=w333, y=w332) -> (x .or. y?=w330:bool)
          }
          frame Enabled {
            n116 = Greater Or Equal?(x=w337, y=w335) -> (x >= y?=w336:bool)
          }
        }
        n117 = Subtract(x=w294, y=w295) -> (x-y=w318:dbl)
        n118 = call "LockedHeading.vi"("LockHeading"=w320, "Heading In"=w297) -> ("LockedHeading"=w296:dbl)  [unwired: 9 in]
        n119 = Divide(x=w318, y=572.75) -> (x/y=w317:dbl)
        n120 = Multiply(x=w319, y=w317) -> (x*y=w316:dbl)
        n121 = In Range and Coerce(upper limit=-0.5, x=w316, lower limit=-1.0) -> (coerced(x)=w293:dbl)  [unwired: 1 out]
        n122 = call "AutonWait.vi"("Target Time (s)"=3.0, "First Time?"=w299) -> ("Completed"=w302:bool)  [unwired: 8 in, 1 out]
        n123 = feedback #5(0.0 ("upper limit")) -> (w305:dbl)
        n124 = Subtract(x=w305, y=0.01) -> (x-y=w306:dbl)
        n125 = In Range and Coerce(upper limit=1.0, x=w293, lower limit=w306) -> (coerced(x)=w290:dbl)  [unwired: 1 out]
        n126 = feedback-in #5(w290) -> ()
        n127 = Or(x=w302, y=w301) -> (x .or. y?=w300:bool)
        n128 = call "IncrementIndex.vi"("Increment?"=w300, "IndexIn"=w324) -> ("IndexOut"=w328:i32)  [unwired: 9 in]
        n129 = call "DriveStraight.vi"("Sensitivity"=0.05, "Range"=w327, "Motor Speed"=w290, "Target"=w296, "Yaw"=w297) -> ("Right"=w323:dbl, "Left"=w322:dbl)  [unwired: 5 in]
        n130 = case shown="False" w300 {
          tunnel: w323 -> [w339 _]
          tunnel: w322 -> [w338 _]
          tunnel: [w339 w340] -> w291
          tunnel: [w338 w340] -> w292
          frame False {
          }
          frame True {
            w340 = 0.0 ("upper limit")
          }
        }
      }
      frame "SlowForward" {
        w379 = 0.25  # Range
        w371 = -1.0  # Motor Speed
        n131 = Index Array(array=w377, index=w376) -> (element=w346:T3)
        n132 = call "EncoderDrive.vi"() -> ("RightEncder"=w347:dbl, "LeftEncoder"=w373:dbl)  [unwired: 10 in]
        n133 = call "GyroActions.vi"("Update?"=FALSE) -> ("Yaw"=w349:dbl)  [unwired: 9 in, 1 out]
        n134 = Not(x=w351) -> (.not. x?=w372:bool)
        n135 = disable-structure shown="Enabled" {
          disable-tunnel: w347 -> [w386 w389]
          disable-tunnel: w373 -> [w383 _]
          disable-tunnel: [w382 w388] -> w353
          disable-tunnel: w346 -> [w381 w387]
          frame Disabled {
            n136 = Greater Or Equal?(x=w383, y=w381) -> (x >= y?=w385:bool)
            n137 = Greater Or Equal?(x=w386, y=w381) -> (x >= y?=w384:bool)
            n138 = Or(x=w385, y=w384) -> (x .or. y?=w382:bool)
          }
          frame Enabled {
            n139 = Greater Or Equal?(x=w389, y=w387) -> (x >= y?=w388:bool)
          }
        }
        n140 = Subtract(x=w346, y=w347) -> (x-y=w370:dbl)
        n141 = call "LockedHeading.vi"("LockHeading"=w372, "Heading In"=w349) -> ("LockedHeading"=w348:dbl)  [unwired: 9 in]
        n142 = Divide(x=w370, y=572.75) -> (x/y=w369:dbl)
        n143 = Multiply(x=w371, y=w369) -> (x*y=w368:dbl)
        n144 = In Range and Coerce(upper limit=-0.65, x=w368, lower limit=-1.0) -> (coerced(x)=w345:dbl)  [unwired: 1 out]
        n145 = call "AutonWait.vi"("Target Time (s)"=4.0, "First Time?"=w351) -> ("Completed"=w354:bool)  [unwired: 8 in, 1 out]
        n146 = feedback #6(0.0 ("upper limit")) -> (w357:dbl)
        n147 = Subtract(x=w357, y=0.01) -> (x-y=w358:dbl)
        n148 = In Range and Coerce(upper limit=1.0, x=w345, lower limit=w358) -> (coerced(x)=w342:dbl)  [unwired: 1 out]
        n149 = feedback-in #6(w342) -> ()
        n150 = Or(x=w354, y=w353) -> (x .or. y?=w352:bool)
        n151 = call "IncrementIndex.vi"("Increment?"=w352, "IndexIn"=w376) -> ("IndexOut"=w380:i32)  [unwired: 9 in]
        n152 = call "DriveStraight.vi"("Sensitivity"=0.05, "Range"=w379, "Motor Speed"=w342, "Target"=w348, "Yaw"=w349) -> ("Right"=w375:dbl, "Left"=w374:dbl)  [unwired: 5 in]
        n153 = case shown="False" w352 {
          tunnel: w375 -> [w391 _]
          tunnel: w374 -> [w390 _]
          tunnel: [w391 w392] -> w343
          tunnel: [w390 w392] -> w344
          frame False {
          }
          frame True {
            w392 = 0.0 ("upper limit")
          }
        }
      }
      frame "HopperDrive" {
        w431 = 0.25  # Range
        w423 = -1.0  # Motor Speed
        n154 = Index Array(array=w429, index=w428) -> (element=w398:T3)
        n155 = call "EncoderDrive.vi"() -> ("RightEncder"=w399:dbl, "LeftEncoder"=w425:dbl)  [unwired: 10 in]
        n156 = call "GyroActions.vi"("Update?"=FALSE) -> ("Yaw"=w401:dbl)  [unwired: 9 in, 1 out]
        n157 = Not(x=w403) -> (.not. x?=w424:bool)
        n158 = disable-structure shown="Enabled" {
          disable-tunnel: w399 -> [w438 w441]
          disable-tunnel: w425 -> [w435 _]
          disable-tunnel: [w434 w439] -> w405
          disable-tunnel: w398 -> [w433 w440]
          frame Disabled {
            n159 = Greater Or Equal?(x=w435, y=w433) -> (x >= y?=w437:bool)
            n160 = Greater Or Equal?(x=w438, y=w433) -> (x >= y?=w436:bool)
            n161 = Or(x=w437, y=w436) -> (x .or. y?=w434:bool)
          }
          frame Enabled {
            n162 = Greater Or Equal?(x=w441, y=w440) -> (x >= y?=w439:bool)
          }
        }
        n163 = Subtract(x=w398, y=w399) -> (x-y=w422:dbl)
        n164 = call "LockedHeading.vi"("LockHeading"=w424, "Heading In"=w401) -> ("LockedHeading"=w400:dbl)  [unwired: 9 in]
        n165 = Divide(x=w422, y=572.75) -> (x/y=w421:dbl)
        n166 = Multiply(x=w423, y=w421) -> (x*y=w420:dbl)
        n167 = In Range and Coerce(upper limit=-0.65, x=w420, lower limit=-1.0) -> (coerced(x)=w397:dbl)  [unwired: 1 out]
        n168 = call "AutonWait.vi"("Target Time (s)"=1.75, "First Time?"=w403) -> ("Completed"=w406:bool)  [unwired: 8 in, 1 out]
        n169 = feedback #7(0.0 ("upper limit")) -> (w409:dbl)
        n170 = Subtract(x=w409, y=0.05) -> (x-y=w410:dbl)
        n171 = In Range and Coerce(upper limit=1.0, x=w397, lower limit=w410) -> (coerced(x)=w396:dbl)  [unwired: 1 out]
        n172 = feedback-in #7(w396) -> ()
        n173 = Or(x=w406, y=w405) -> (x .or. y?=w404:bool)
        n174 = call "IncrementIndex.vi"("Increment?"=w404, "IndexIn"=w428) -> ("IndexOut"=w432:i32)  [unwired: 9 in]
        n175 = call "DriveStraight.vi"("Sensitivity"=0.05, "Range"=w431, "Motor Speed"=w396, "Target"=w400, "Yaw"=w401) -> ("Right"=w427:dbl, "Left"=w426:dbl)  [unwired: 5 in]
        n176 = case shown="False" w404 {
          tunnel: w427 -> [w443 _]
          tunnel: w426 -> [w442 _]
          tunnel: [w443 w444] -> w394
          tunnel: [w442 w444] -> w395
          frame False {
          }
          frame True {
            w444 = 0.0 ("upper limit")
          }
        }
      }
      frame "StraightBack" {
        w474 = 0.25  # Range
        w461 = 0.85  # Motor Speed
        n177 = Index Array(array=w471, index=w470) -> (element=w447:T3)
        n178 = call "GyroActions.vi"("Update?"=FALSE) -> ("Yaw"=w450:dbl)  [unwired: 9 in, 1 out]
        n179 = call "EncoderDrive.vi"() -> ("RightEncder"=w448:dbl, "LeftEncoder"=w468:dbl)  [unwired: 10 in]
        n180 = call "LockedHeading.vi"("LockHeading"=TRUE, "Heading In"=w450) -> ("LockedHeading"=w449:dbl)  [unwired: 9 in]
        n181 = disable-structure shown="Enabled" {
          disable-tunnel: w448 -> [w480 w483]
          disable-tunnel: w468 -> [w477 _]
          disable-tunnel: [w476 w481] -> w463
          disable-tunnel: w447 -> [w475 w482]
          frame Disabled {
            n182 = Less Or Equal?(x=w477, y=w475) -> (x <= y?=w479:bool)
            n183 = Less Or Equal?(x=w480, y=w475) -> (x <= y?=w478:bool)
            n184 = Or(x=w479, y=w478) -> (x .or. y?=w476:bool)
          }
          frame Enabled {
            n185 = Less Or Equal?(x=w483, y=w482) -> (x <= y?=w481:bool)
          }
        }
        n186 = Subtract(x=w447, y=w448) -> (x-y=w469:dbl)
        n187 = Divide(x=w469, y=w447) -> (x/y=w462:dbl)
        n188 = Multiply(x=w461, y=w462) -> (x*y=w460:dbl)
        n189 = In Range and Coerce(upper limit=1.0, x=w460, lower limit=0.5) -> (coerced(x)=w459:dbl)  [unwired: 1 out]
        n190 = call "DriveStraight.vi"("Reverse?"=TRUE, "Sensitivity"=0.05, "Range"=w474, "Motor Speed"=w459, "Target"=w449, "Yaw"=w450) -> ("Right"=w466:dbl, "Left"=w467:dbl)  [unwired: 4 in]
        n191 = call "IncrementIndex.vi"("Increment?"=w463, "IndexIn"=w470) -> ("IndexOut"=w472:i32)  [unwired: 9 in]
        n192 = case shown="False" w463 {
          tunnel: w466 -> [w484 _]
          tunnel: w467 -> [w485 _]
          tunnel: [w484 w486] -> w464
          tunnel: [w485 w486] -> w465
          frame False {
          }
          frame True {
            w486 = 0.0 ("upper limit")
          }
        }
      }
      frame "SolenoidControl" {
        w489 = 0.0 ("Yaw")
        w497 = 0.0 ("Left")
        n193 = Index Array(array=w500, index=w496) -> (element=w498:bool)
        n194 = Index Array(array=w499, index=w496) -> (element=w494:bool)
        n195 = call "FuelFlap.vi"("Fuel Flap"=w494) -> ()  [unwired: 11 in]
        n196 = call "GearFlap.vi"("Gear Flap"=w494) -> ()  [unwired: 11 in]
        n197 = call "GearLift.vi"("Gear Up"=w498) -> ()  [unwired: 11 in]
        n198 = call "IncrementIndex.vi"("Increment?"=w495, "IndexIn"=w496) -> ("IndexOut"=w501:i32)  [unwired: 9 in]
      }
      frame "GradLeftCurve" {
        w504 = 0.0 ("Yaw")
        w507 = 0.0 ("Power")
        w509 = 0.0 ("Left")
        n199 = call "GyroActions.vi"("Update?"=FALSE) -> ("Yaw"=w505:dbl)  [unwired: 9 in, 1 out]
        n200 = Less Or Equal?(x=w505, y=-45.0) -> (x <= y?=w510:bool)
        n201 = call "IncrementIndex.vi"("Increment?"=w510, "IndexIn"=w514) -> ("IndexOut"=w513:i32)  [unwired: 9 in]
      }
      frame "GradRightCurve" {
        w517 = 0.0 ("Yaw")
        w520 = 0.0 ("Power")
        w522 = 0.0 ("Left")
        n202 = call "GyroActions.vi"("Update?"=FALSE) -> ("Yaw"=w518:dbl)  [unwired: 9 in, 1 out]
        n203 = Less Or Equal?(x=w518, y=45.0) -> (x <= y?=w523:bool)
        n204 = call "IncrementIndex.vi"("Increment?"=w523, "IndexIn"=w527) -> ("IndexOut"=w526:i32)  [unwired: 9 in]
      }
      frame "TurnLeft90" {
        w534 = 0.0 ("Power")
        w531 = -90.0  # Target Position
        w542 = 65.0  # Slow Range
        w543 = 1.0  # Motor Power In
        w544 = 0.25  # Target Range
        w545 = 0.24  # Min Power
        n205 = call "GyroActions.vi"("Update?"=FALSE) -> ("Yaw"=w532:dbl)  [unwired: 9 in, 1 out]
        n206 = call "TurnSmooth.vi"("Min Power"=w545, "First Time?"=w540, "Target Range"=w544, "Current Position"=w532, "Target Position"=w531, "Slow Range"=w542, "Motor Power In"=w543) -> ("Done"=w541:bool, "Right Motor Power"=w535:dbl, "Left Motor Power"=w536:dbl)  [unwired: 2 in]
        n207 = call "IncrementIndex.vi"("Increment?"=w541, "IndexIn"=w539) -> ("IndexOut"=w538:i32)  [unwired: 9 in]
      }
      frame "SharpLeftCurve" {
        w553 = 0.0 ("Power")
        w550 = -90.0  # Target Position
        w560 = 30.0  # Slow Range
        w561 = 1.0  # Motor Power In
        w562 = 0.25  # Target Range
        w563 = 0.24  # Min Power
        n208 = call "GyroActions.vi"("Update?"=FALSE) -> ("Yaw"=w551:dbl)  [unwired: 9 in, 1 out]
        n209 = call "TurnSmooth.vi"("Min Power"=w563, "First Time?"=w558, "Target Range"=w562, "Current Position"=w551, "Target Position"=w550, "Slow Range"=w560, "Motor Power In"=w561) -> ("Done"=w559:bool, "Right Motor Power"=w554:dbl)  [unwired: 2 in, 1 out]
        n210 = call "IncrementIndex.vi"("Increment?"=w559, "IndexIn"=w557) -> ("IndexOut"=w556:i32)  [unwired: 9 in]
      }
      frame "TurnRight90" {
        w570 = 0.0 ("Power")
        w567 = 90.0  # Target Position
        w574 = 65.0  # Slow Range
        w575 = 1.0  # Motor Power In
        w576 = 0.25  # Target Range
        w577 = 0.3  # Min Power
        n211 = call "GyroActions.vi"("Update?"=FALSE) -> ("Yaw"=w568:dbl)  [unwired: 9 in, 1 out]
        n212 = call "TurnSmooth.vi"("Min Power"=w577, "First Time?"=w581, "Target Range"=w576, "Current Position"=w568, "Target Position"=w567, "Slow Range"=w574, "Motor Power In"=w575) -> ("Done"=w578:bool, "Right Motor Power"=w571:dbl, "Left Motor Power"=w572:dbl)  [unwired: 2 in]
        n213 = call "IncrementIndex.vi"("Increment?"=w578, "IndexIn"=w579) -> ("IndexOut"=w580:i32)  [unwired: 9 in]
      }
      frame "SharpRightCurve" {
        w589 = 0.0 ("Power")
        w586 = 90.0  # Target Position
        w592 = 65.0  # Slow Range
        w593 = 1.0  # Motor Power In
        w594 = 0.25  # Target Range
        w595 = 0.3  # Min Power
        n214 = call "GyroActions.vi"("Update?"=FALSE) -> ("Yaw"=w587:dbl)  [unwired: 9 in, 1 out]
        n215 = call "TurnSmooth.vi"("Min Power"=w595, "First Time?"=w599, "Target Range"=w594, "Current Position"=w587, "Target Position"=w586, "Slow Range"=w592, "Motor Power In"=w593) -> ("Done"=w596:bool, "Left Motor Power"=w590:dbl)  [unwired: 2 in, 1 out]
        n216 = call "IncrementIndex.vi"("Increment?"=w596, "IndexIn"=w597) -> ("IndexOut"=w598:i32)  [unwired: 9 in]
      }
      frame "TurnLeft60" {
        w606 = 0.0 ("Power")
        w603 = -60.0  # Target Position
        w614 = 55.0  # Slow Range
        w615 = 1.0  # Motor Power In
        w616 = 0.25  # Target Range
        w617 = 0.23  # Min Power
        n217 = call "GyroActions.vi"("Update?"=FALSE) -> ("Yaw"=w604:dbl)  [unwired: 9 in, 1 out]
        n218 = call "TurnSmooth.vi"("Min Power"=w617, "First Time?"=w611, "Target Range"=w616, "Current Position"=w604, "Target Position"=w603, "Slow Range"=w614, "Motor Power In"=w615) -> ("Done"=w610:bool, "Right Motor Power"=w607:dbl, "Left Motor Power"=w608:dbl)  [unwired: 2 in]
        n219 = call "IncrementIndex.vi"("Increment?"=w610, "IndexIn"=w613) -> ("IndexOut"=w612:i32)  [unwired: 9 in]
      }
      frame "TurnRight60" {
        w624 = 0.0 ("Power")
        w621 = 60.0  # Target Position
        w632 = 55.0  # Slow Range
        w633 = 1.0  # Motor Power In
        w634 = 0.25  # Target Range
        w635 = 0.16  # Min Power
        n220 = call "GyroActions.vi"("Update?"=FALSE) -> ("Yaw"=w622:dbl)  [unwired: 9 in, 1 out]
        n221 = call "TurnSmooth.vi"("Min Power"=w635, "First Time?"=w630, "Target Range"=w634, "Current Position"=w622, "Target Position"=w621, "Slow Range"=w632, "Motor Power In"=w633) -> ("Done"=w631:bool, "Right Motor Power"=w625:dbl, "Left Motor Power"=w626:dbl)  [unwired: 2 in]
        n222 = call "IncrementIndex.vi"("Increment?"=w631, "IndexIn"=w629) -> ("IndexOut"=w628:i32)  [unwired: 9 in]
      }
      frame "TurnLeft45" {
        w642 = 0.0 ("Power")
        w639 = -70.0  # Target Position
        w650 = 55.0  # Slow Range
        w651 = 1.0  # Motor Power In
        w652 = 0.25  # Target Range
        w653 = 0.23  # Min Power
        n223 = call "GyroActions.vi"("Update?"=FALSE) -> ("Yaw"=w640:dbl)  [unwired: 9 in, 1 out]
        n224 = call "TurnSmooth.vi"("Min Power"=w653, "First Time?"=w648, "Target Range"=w652, "Current Position"=w640, "Target Position"=w639, "Slow Range"=w650, "Motor Power In"=w651) -> ("Done"=w649:bool, "Right Motor Power"=w643:dbl, "Left Motor Power"=w644:dbl)  [unwired: 2 in]
        n225 = call "IncrementIndex.vi"("Increment?"=w649, "IndexIn"=w647) -> ("IndexOut"=w646:i32)  [unwired: 9 in]
      }
      frame "TurnRight45" {
        w660 = 0.0 ("Power")
        w657 = 65.0  # Target Position
        w668 = 55.0  # Slow Range
        w669 = 1.0  # Motor Power In
        w670 = 0.25  # Target Range
        w671 = 0.23  # Min Power
        n226 = call "GyroActions.vi"("Update?"=FALSE) -> ("Yaw"=w658:dbl)  [unwired: 9 in, 1 out]
        n227 = call "TurnSmooth.vi"("Min Power"=w671, "First Time?"=w666, "Target Range"=w670, "Current Position"=w658, "Target Position"=w657, "Slow Range"=w668, "Motor Power In"=w669) -> ("Done"=w667:bool, "Right Motor Power"=w661:dbl, "Left Motor Power"=w662:dbl)  [unwired: 2 in]
        n228 = call "IncrementIndex.vi"("Increment?"=w667, "IndexIn"=w665) -> ("IndexOut"=w664:i32)  [unwired: 9 in]
      }
      frame "Shoot" {
        w674 = 0.0 ("Yaw")
        w684 = 0.0 ("Left")
        n229 = call "AutonWait.vi"("Target Time (s)"=8.0, "First Time?"=w680) -> ("Completed"=w679:bool)  [unwired: 8 in, 1 out]
        n230 = call "IncrementIndex.vi"("Increment?"=w679, "IndexIn"=w683) -> ("IndexOut"=w682:i32)  [unwired: 9 in]
      }
      frame "ShortShoot" {
        w687 = 0.0 ("Yaw")
        w700 = 0.0 ("Left")
        n231 = call "AutonWait.vi"("Target Time (s)"=8.0, "First Time?"=w696) -> ("ElapsedTime"=w689:dbl, "Completed"=w691:bool)  [unwired: 8 in]
        n232 = Greater Or Equal?(x=w689, y=2.0) -> (x >= y?=w690:bool)
        n233 = case shown="True" w690 {
          tunnel: [0.0 ("RearMotorIn") 1.0 ("RearMotorIn")] -> w695
          tunnel: [WPI_RelayValue."Off" ("RelayValue") WPI_RelayValue."Forward" ("RelayValue")] -> w694
          frame False {
          }
          frame True {
          }
        }
        n234 = call "IncrementIndex.vi"("Increment?"=w691, "IndexIn"=w699) -> ("IndexOut"=w698:i32)  [unwired: 9 in]
      }
      frame "SpinUp" {
        w707 = 0.0 ("Yaw")
        w710 = 1.0 ("RearMotorIn")
        w716 = 0.0 ("Left")
        n235 = call "AutonWait.vi"("Target Time (s)"=3.0, "First Time?"=w712) -> ("Completed"=w711:bool)  [unwired: 8 in, 1 out]
        n236 = call "IncrementIndex.vi"("Increment?"=w711, "IndexIn"=w715) -> ("IndexOut"=w714:i32)  [unwired: 9 in]
      }
      frame "Wait" {
        w719 = 0.0 ("Yaw")
        w722 = 0.0 ("RearMotorIn")
        w723 = 0.0 ("Left")
        n237 = call "AutonWait.vi"("Target Time (s)"=1.3, "First Time?"=w728) -> ("Completed"=w724:bool)  [unwired: 8 in, 1 out]
        n238 = call "IncrementIndex.vi"("Increment?"=w724, "IndexIn"=w726) -> ("IndexOut"=w725:i32)  [unwired: 9 in]
      }
      frame "VisionTarget" {
        n239 = call "GyroActions.vi"() -> ("Yaw"=w733:dbl)  [unwired: 10 in, 1 out]
        n240 = call "VisionMode.vi"() -> ("ModeOut"=w738:string)  [unwired: 3 in]
        n241 = Select(t="Init", s=w739, f=w738) -> (s? t:f=w737:string)
        n242 = case shown="\"Init\", Default" w737 {
          tunnel: [w753 w758 w775 w793 w806] -> w746
          tunnel: [w753 w758 w775 w792 w806] -> w745
          tunnel: [0.0 ("Power") 0.0 ("Power") 0.0 ("Power") 0.0 ("Power") 0.0 ("Power")] -> w744
          tunnel: [WPI_RelayValue."Off" ("RelayValue") WPI_RelayValue."Off" ("RelayValue") WPI_RelayValue."Off" ("RelayValue") WPI_RelayValue."Off" ("RelayValue") WPI_RelayValue."Off" ("RelayValue")] -> w743
          tunnel: [TRUE _ _ _ _] -> w742
          tunnel: w741 -> [w751 w757 w774 w789 w804]
          tunnel: [w750 w757 w774 w789 w804] -> w740
          tunnel: [0.0 ("LockedHeading") 0.0 ("LockedHeading") w766 w787 w803] -> w732
          frame "Stop" {
            w753 = 0.0 ("Power")
            n243 = call "VisionMode.vi"("ModeIn"="Stop") -> ()  [unwired: 2 in, 1 out]
            n244 = call "IncrementIndex.vi"("Increment?"=TRUE, "IndexIn"=w751) -> ("IndexOut"=w750:i32)  [unwired: 9 in]
          }
          frame "Init", Default {
            w758 = 0.0 ("Motor Power Out")
            w762 = 0.0 ("CenterXIn")
            w763 = TRUE ("Input")
            n245 = call "GyroActions.vi"("Zero"=TRUE) -> ()  [unwired: 9 in, 2 out]
            n246 = call "TargetCoord.vi"("CenterXIn"=w762, "CenterYIn"=w762, "ScoreIn"=w762, "Update?"=TRUE) -> ()  [unwired: 13 in, 3 out]
            n247 = call "FirstTime"("Update?"=w763, "Input"=w763) -> ()  [unwired: 3 in, 1 out]
            n248 = call "VisionMode.vi"("ModeIn"="Acquire") -> ()  [unwired: 2 in, 1 out]
          }
          frame "Acquire" {
            w775 = 0.0 ("Power")
            w781 = TRUE ("EnableVision")
            n249 = call "TargetCoord.vi"() -> ("CenterXOut"=w771:dbl, "Target?"=w768:bool)  [unwired: 17 in, 1 out]
            n250 = call "EnableVision.vi"("Update"=w781, "EnableVision"=w781) -> ()  [unwired: 8 in, 2 out]
            n251 = feedback-in #8(w771) -> ()
            n252 = feedback #8() -> (w770:dbl)  [unwired: 1 in]
            n253 = Not Equal?(x=w771, y=w770) -> (x != y?=w769:bool)
            n254 = And(x=w769, y=w768) -> (x .and. y?=w767:bool)
            n255 = call "CameraAngleMath.vi"("TargetXCenter"=w771) -> ("TargetAngle"=w772:dbl)  [unwired: 10 in]
            n256 = Select(t="Move" ("ModeIn"), s=w767, f="Acquire" ("ModeIn")) -> (s? t:f=w780:string)
            n257 = Add(x=w772, y=0.5) -> (x+y=w766:dbl)
            n258 = call "VisionMode.vi"("ModeIn"=w780) -> ()  [unwired: 2 in, 1 out]
            n259 = call "LockedHeading.vi"("LockHeading"=FALSE, "Heading In"=w766) -> ()  [unwired: 9 in, 1 out]
          }
          frame "Move" {
            n260 = call "EnableVision.vi"("Update"=TRUE ("EnableVision")) -> ()  [unwired: 9 in, 2 out]
            n261 = call "LockedHeading.vi"("LockHeading"=TRUE) -> ("LockedHeading"=w787:dbl)  [unwired: 10 in]
            n262 = call "GyroActions.vi"("Update?"=FALSE) -> ("Yaw"=w801:dbl)  [unwired: 9 in, 1 out]
            n263 = call "FirstTime"() -> ("Output"=w788:bool)  [unwired: 5 in]
            n264 = call "TurnSmooth.vi"("Min Power"=0.2, "First Time?"=w788, "Target Range"=0.5, "Current Position"=w801, "Target Position"=w787, "Slow Range"=45.0, "Motor Power In"=1.0) -> ("Done"=w800:bool, "Right Motor Power"=w792:dbl, "Left Motor Power"=w793:dbl)  [unwired: 2 in]
            n265 = Select(t="Check", s=w800, f="Move") -> (s? t:f=w797:string)
            n266 = call "FirstTime"("Update?"=TRUE, "Input"=w800) -> ()  [unwired: 3 in, 1 out]
            n267 = call "VisionMode.vi"("ModeIn"=w797) -> ()  [unwired: 2 in, 1 out]
          }
          frame "Check" {
            w806 = 0.0 ("Power")
            n268 = call "GyroActions.vi"("Update?"=FALSE) -> ("Yaw"=w818:dbl)  [unwired: 9 in, 1 out]
            n269 = call "LockedHeading.vi"("LockHeading"=TRUE) -> ("LockedHeading"=w803:dbl)  [unwired: 10 in]
            n270 = feedback #9(TRUE ("Completed")) -> (w814:bool)
            n271 = call "Wait.vi"("Target Time (s)"=0.2 ("Target Time"), "First Time?"=w814) -> ("Completed"=w809:bool)  [unwired: 9 in]
            n272 = feedback-in #9(w809) -> ()
            n273 = Subtract(x=w818, y=w803) -> (x-y=w817:dbl)
            n274 = Absolute Value(x=w817) -> (abs(x)=w816:dbl)
            n275 = Less?(x=w816, y=0.5) -> (x < y?=w810:bool)
            n276 = And(x=w809, y=w810) -> (x .and. y?=w811:bool)
            n277 = Select(t="Stop", s=w811, f="Move") -> (s? t:f=w820:string)
            n278 = call "VisionMode.vi"("ModeIn"=w820) -> ()  [unwired: 2 in, 1 out]
          }
        }
      }
      frame "Pause" {
        w833 = 0.0 ("Yaw")
        w836 = 0.0 ("Power")
        n279 = Index Array(array=w831, index=w830) -> (element=w825:T3)
        n280 = call "AutonWait.vi"("Target Time (s)"=0.75, "First Time?"=w839) -> ("Completed"=w837:bool)  [unwired: 8 in, 1 out]
        n281 = call "IncrementIndex.vi"("Increment?"=w837, "IndexIn"=w830) -> ("IndexOut"=w838:i32)  [unwired: 9 in]
        n282 = Equal?(x=T3 1, y=w825) -> (x = y?=w828:bool)
        n283 = Select(t=1.0, s=w828, f=0.0) -> (s? t:f=w824:dbl)
      }
    }
    n284 = call "AutonTxtFile.vi"("dataName"="Current Gyro", "mode"=T10."Float", "float"=w48, "string"=w32) -> ("flowControl"=w40:string)  [unwired: 10 in, 1 out]
    n285 = call "AutonTxtFile.vi"("dataName"="Target Angle", "mode"=T10."Float", "float"=w39, "string"=w40) -> ("flowControl"=w38:string)  [unwired: 10 in, 1 out]
    n286 = call "AutonTxtFile.vi"("dataName"="Right Encoder", "mode"=T10."Float", "float"=w45, "string"=w38) -> ("flowControl"=w36:string)  [unwired: 10 in, 1 out]
    n287 = call "AutonTxtFile.vi"("dataName"="Encoder Target", "mode"=T10."Integer", "integer"=w37, "string"=w36) -> ("flowControl"=w35:string)  [unwired: 10 in, 1 out]
    n288 = call "Feeder.vi"("Power"=w78) -> ()  [unwired: 11 in]
    n289 = call "StirSticks.vi"("RelayValue"=w77) -> ()  [unwired: 11 in]
    n290 = call "Intake.vi"("Power"=w31) -> ()  [unwired: 11 in]
    n291 = call "Shooter.vi"("FrontMotorIn"=w51, "Control Mode"=WPI_CANTalonSRX_APIControlMode."Speed", "RearMotorIn"=w53) -> ()  [unwired: 1 in]
    n292 = call "AutonTxtFile.vi"("dataName"="Left Drive Motor", "mode"=T10."Float", "float"=w63, "string"=w35) -> ("flowControl"=w59:string)  [unwired: 10 in, 1 out]
    n293 = call "AutonTxtFile.vi"("dataName"="Right Drive Motor", "mode"=T10."Float", "float"=w60, "string"=w59) -> ("flowControl"=w54:string)  [unwired: 10 in, 1 out]
    n294 = call "AutonTxtFile.vi"("dataName"="Rear Shooter Speed", "mode"=T10."Float", "float"=w53, "string"=w54) -> ("flowControl"=w52:string)  [unwired: 10 in, 1 out]
    n295 = call "AutonTxtFile.vi"("dataName"="Front Shooter Speed", "mode"=T10."Float", "float"=w51, "string"=w52, "newLine?"=TRUE) -> ()  [unwired: 9 in, 2 out]
    n296 = call <vilib>:"WPI_MotorControlSetOutput.vi"("Output"=w63, "MotorControlDevRef"=w75) -> ()  [unwired: 7 in, 3 out]
    n297 = call <vilib>:"WPI_MotorControlSetOutput.vi"("Output"=w60, "MotorControlDevRef"=w74) -> ()  [unwired: 7 in, 3 out]
    n298 = Wait (ms)(milliseconds to wait=u32 5) -> ()  [unwired: 1 out]
  }
